vi "Demo2.vi"() -> ()   [LabVIEW 2014]
uses:
  1/ExampleClass.lvclass
  2/ExampleClass2.lvclass
  1/ExampleClass.lvclass/ExampleClass.ctl
  2/ExampleClass2.lvclass/ExampleClass2.ctl
  Singleton/Singleton.lvclass
panel:
  in  "stop":bool
  out "Numeric 3":dbl
  out "Numeric 2":dbl
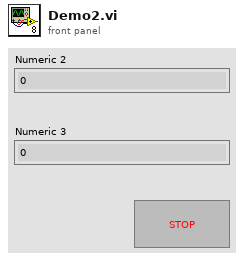
[diagram p1: front panel]
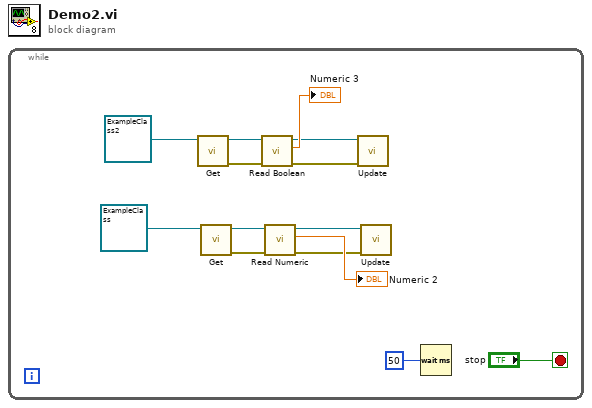
[diagram p0: block diagram]
diagram:
  n1 = while {
    stop <- "stop" stop-if-true
    n2 = call "Get.vi"("Template"=refnum<class "ExampleClass2.lvclass"> refnum ("ExampleClass2")) -> ("error out"=w2:errorcluster, "object"=w1:refnum<class "ExampleClass2.lvclass">)  [unwired: 9 in]
    n3 = call "Get.vi"("Template"=refnum<class "ExampleClass.lvclass"> refnum ("ExampleClass")) -> ("error out"=w4:errorcluster, "object"=w3:refnum<class "ExampleClass.lvclass">)  [unwired: 9 in]
    n4 = call "Read Boolean.vi"("error in (no error)"=w2, "ExampleClass2 in"=w1) -> ("error out"=w10:errorcluster, "Numeric"=→"Numeric 3":dbl, "ExampleClass2 out"=w9:refnum<class "ExampleClass2.lvclass">)  [unwired: 7 in]
    n5 = call "Read Numeric.vi"("error in (no error)"=w4, "ExampleClass in"=w3) -> ("error out"=w5:errorcluster, "Numeric"=→"Numeric 2":dbl, "ExampleClass out"=w6:refnum<class "ExampleClass.lvclass">)  [unwired: 7 in]
    n6 = call "Update.vi"("error in (no error)"=w10, "Object"=w9) -> ()  [unwired: 8 in, 2 out]
    n7 = call "Update.vi"("error in (no error)"=w5, "Object"=w6) -> ()  [unwired: 8 in, 2 out]
    n8 = Wait (ms)(milliseconds to wait=u32 50) -> ()  [unwired: 1 out]
  }
